vi "Get Result.vi"(8 "error in (no error)":errorcluster, 11 "Pulse Driver in":refnum<class "Pulse Driver.lvclass">) -> (0 "error out":errorcluster, 2 "Result":refnum<class "Acquired Result.lvclass">, 3 "Pulse Driver out":refnum<class "Pulse Driver.lvclass">)   [LabVIEW 2016, in "Pulse Driver.lvclass"]
uses:
  Pulse Driver.lvclass
  Results/Acquired Result/Acquired Result.lvclass
  Pulse Driver.lvclass/Pulse Driver.ctl
  Results/Acquired Result/Acquired Result.lvclass/Acquired Result.ctl
  Results/Acquired Result/Write Final.vi
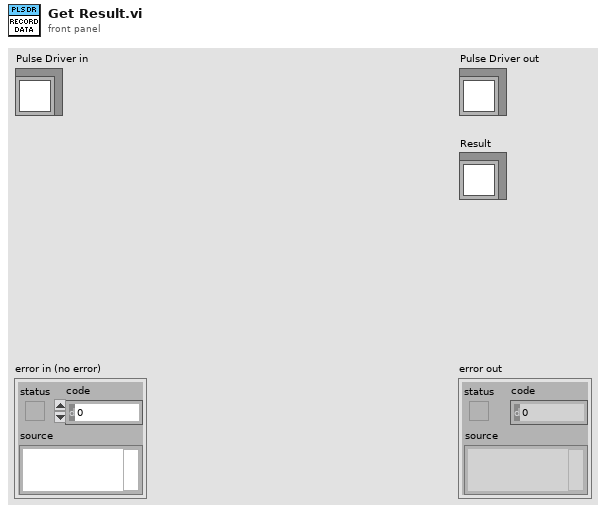
[diagram p1: front panel]
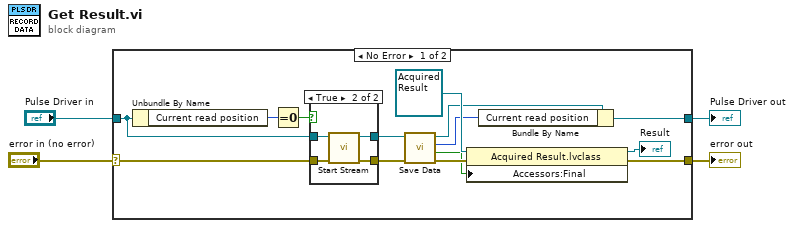
[diagram p0: block diagram]
diagram:
  n1 = case shown="No Error" "error in (no error)" {
    selector: "error in (no error)" -> [w16 w26]
    tunnel: [w11 w26] -> w3
    tunnel: [w15 w25] -> w1
    tunnel: "Pulse Driver in" -> [w14 w25]
    frame No Error {
      n2 = Unbundle By Name(w14) -> ("Current read position"=w18:i32)
      n3 = Equal To 0?(x=w18) -> (x = 0?=w17:bool)
      n4 = case shown="True" w17 {
        tunnel: w14 -> [w19 w23]
        tunnel: w16 -> [w20 w22]
        tunnel: [w20 w24] -> w10
        tunnel: [w19 w21] -> w5
        frame False {
        }
        frame True {
          n5 = call-dynamic "Start Stream.vi"("error in (no error)"=w22, "Pulse Driver in"=w23) -> ("error out"=w24:errorcluster, "Pulse Driver out"=w21:refnum<class "Pulse Driver.lvclass">)  [unwired: 8 in]
        }
      }
      n6 = call-dynamic "Save Data.vi"("error in (no error)"=w10, "Pulse Driver in"=w5) -> ("error out"=w8:errorcluster, "Finished"=w7:bool, "Current read position"=w6:i32, "Pulse Driver out"=w9:refnum<class "Pulse Driver.lvclass">)  [unwired: 6 in]
      n7 = property class="Acquired Result.lvclass"(reference=refnum<class "Acquired Result.lvclass"> refnum ("Result"), error in=w8, "Accessors:Final"=w7) -> (reference out=→"Result":refnum<class "Acquired Result.lvclass">, error out=w11:errorcluster)
      n8 = Bundle By Name(cluster=w9, "Current read position"=w6) -> (w15:refnum<class "Pulse Driver.lvclass">)
    }
    frame Error {
    }
  }
  "error out" <- w3
  "Pulse Driver out" <- w1
